vi "Motors Datum Position.vi"(7 "error in":errorcluster, 8 "VISA in":refnum<visa-resource-name>, 9 "Axis":i32) -> (0 "error out":errorcluster, 1 "VISA out":refnum<visa-resource-name>, 3 "Datum Position (steps)":string)   [LabVIEW 2018]
panel:
  out "number of replacements 2":i32
  out "number of replacements":i32
  out "QP buffer":string
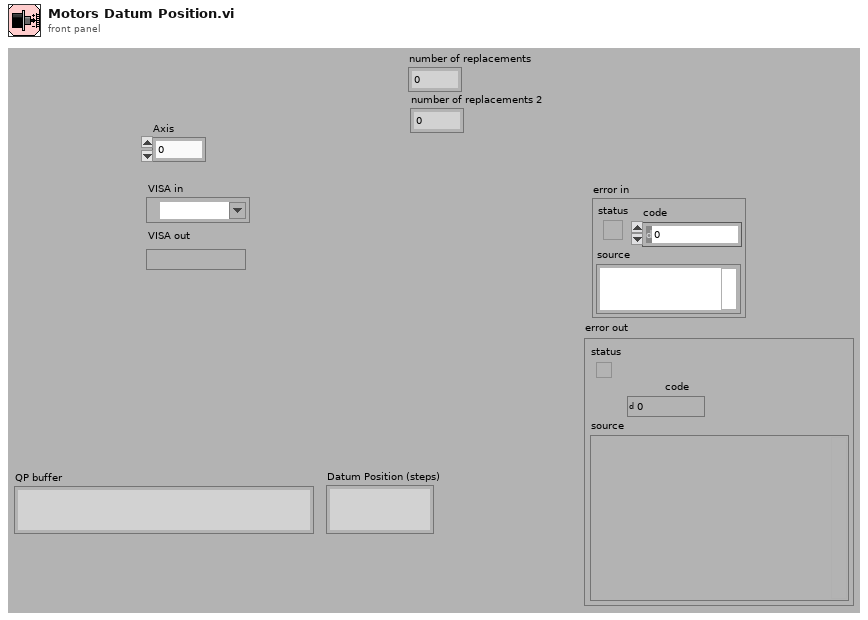
[diagram p1: front panel]
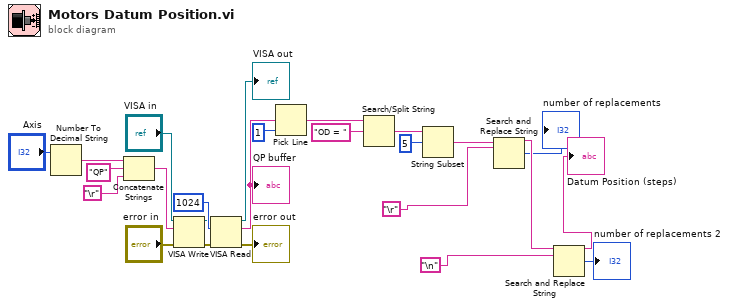
[diagram p0: block diagram]
diagram:
  n1 = Number To Decimal String(number="Axis") -> (decimal integer string=w21:string)  [unwired: 1 in]
  n2 = Concatenate Strings(w21, "QP" ("Initial command 1"), "\r") -> (w20:string)
  n3 = VISA Write(VISA resource name="VISA in", write buffer=w20, error in (no error)="error in") -> (VISA resource name out=w19:refnum<visa-resource-name>, error out=w18:errorcluster)  [unwired: 1 out]
  n4 = VISA Read(VISA resource name=w19, byte count=u32 1024, error in (no error)=w18) -> (VISA resource name out=→"VISA out":refnum<visa-resource-name>, read buffer=w16:string, error out=→"error out":errorcluster)  [unwired: 1 out]
  "QP buffer" <- w16
  n5 = Pick Line(multi-line string=w16, line index=1) -> (output string=w12:string)  [unwired: 1 in]
  n6 = Search/Split String(string=w12, search string/char (-)="OD = ") -> (match + rest of string=w10:string)  [unwired: 1 in, 2 out]
  n7 = String Subset(string=w10, offset (0)=5) -> (substring=w7:string)  [unwired: 1 in]
  n8 = Search and Replace String(input string=w7, search string="\r") -> (result string=w5:string, number of replacements=→"number of replacements":i32)  [unwired: 6 in, 2 out]
  n9 = Search and Replace String(input string=w5, search string="\n") -> (result string=→"Datum Position (steps)":string, number of replacements=→"number of replacements 2":i32)  [unwired: 6 in, 2 out]
